vi "Index Array (String).vi"(8 "error in (no error)":errorcluster, 9 "index":i32, 10 "JSON Value in":refnum<class "JSON Value.lvclass">) -> (0 "error out":errorcluster, 1 "String":string)   [LabVIEW 2016, in "JSON Value.lvclass"]
doc: "Returns the String value of the JSON String element of the JSON array at index."
uses:
  JSON Value.lvclass
  Read Value/Read value (String).vi
  Index Array (Value).vi
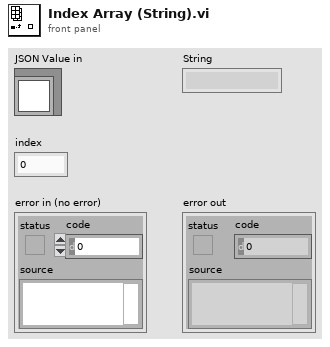
[diagram p1: front panel]
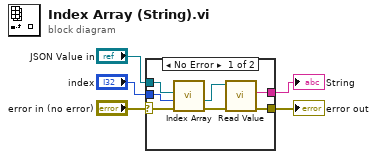
[diagram p0: block diagram]
diagram:
  n1 = case shown="No Error" "error in (no error)" {
    selector: "error in (no error)" -> [w9 w13]
    tunnel: [w10 w13] -> w4
    tunnel: "JSON Value in" -> [w8 _]
    tunnel: "index" -> [w7 _]
    tunnel: [w11 _] -> w1
    frame No Error {
      n2 = call-poly "Index Array.vi"("error in"=w9, "index"=w7, "JSON Value in"=w8) -> ("error out"=w12:errorcluster, "JSON Value out"=w6:refnum<class "JSON Value.lvclass">)  [unwired: 7 in]
      n3 = call-poly "Read Value.vi"("error in (no error)"=w12, "JSON String in"=w6) -> ("error out"=w10:errorcluster, "value"=w11:string)  [unwired: 8 in]
    }
    frame Error {
    }
  }
  "error out" <- w4
  "String" <- w1
